vi "push array double.vi"(0 "Array":dbl[](array[numeric]), 2 "mode":enum16{"forwards (i=0)", "backwards (i=n)"}(ring), 11 "Element":dbl) -> (8 "Array out":dbl[](array[numeric]))   [LabVIEW 2010]
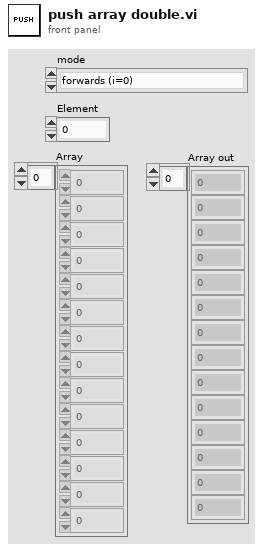
[diagram p1: front panel]
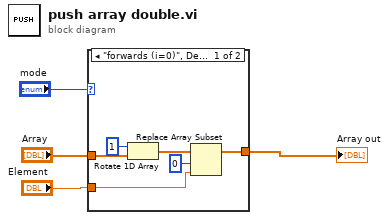
[diagram p0: block diagram]
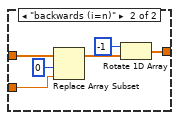
[diagram p2: hidden frame]
diagram:
  n1 = case shown="\"forwards (i=0)\", Default" "mode" {
    tunnel: "Array" -> [w10 w15]
    tunnel: "Element" -> [w7 w14]
    tunnel: [w5 w11] -> w1
    frame "forwards (i=0)", Default {
      n2 = Rotate 1D Array(1:w10, 2:1 ("n")) -> (0:w8:dbl[])
      n3 = Replace Array Subset(array=w8, new element=w7, index=0 ("Index")) -> (w5:dbl[])
    }
    frame "backwards (i=n)" {
      n4 = Replace Array Subset(array=w15, new element=w14, index=0 ("Index")) -> (w12:dbl[])
      n5 = Rotate 1D Array(1:w12, 2:-1 ("n")) -> (0:w11:dbl[])
    }
  }
  "Array out" <- w1
